vi "Page Log.vi"() -> ()   [LabVIEW 2018, in "Main.lvlib"]
uses:
  Main.lvlib
panel:
  out "current time":timestamp
  in  "Listbox":i32(listbox)=-1
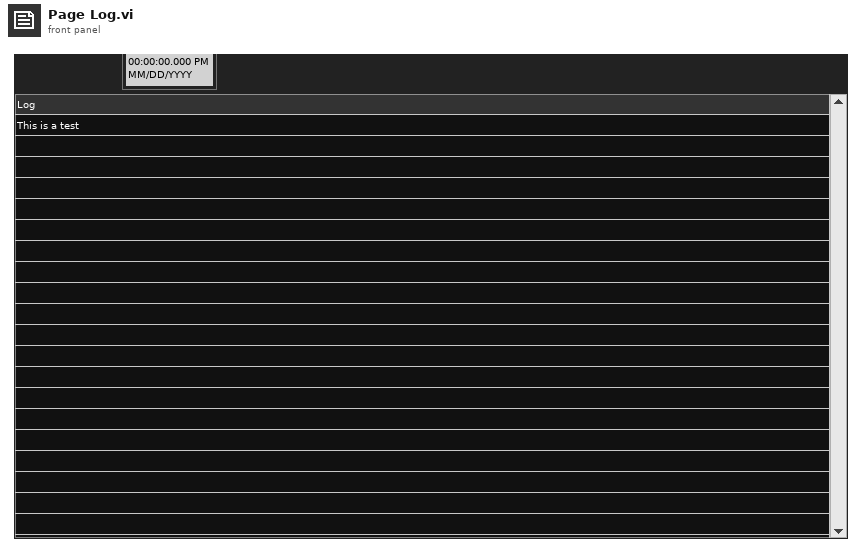
[diagram p1: front panel]
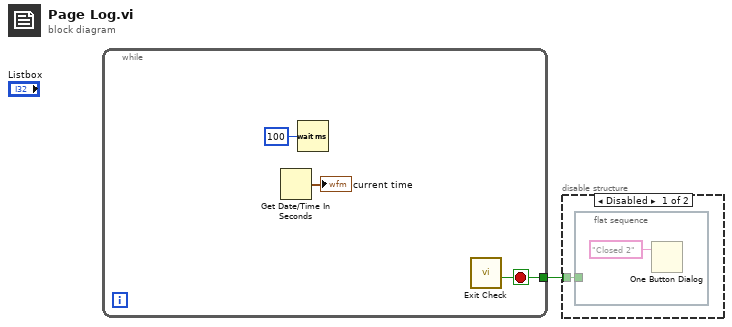
[diagram p0: block diagram]
diagram:
  n1 = while {
    tunnel: [w2] -> w1
    stop <- w2 stop-if-true
    n2 = Get Date/Time In Seconds() -> (seconds since 1Jan1904=→"current time":timestamp)
    n3 = Wait (ms)(milliseconds to wait=u32 100) -> ()  [unwired: 1 out]
    n4 = call "Exit Check.vi"() -> ("Exit?"=w2:bool)  [unwired: 10 in, 1 out]
  }
  n5 = disable-structure shown="Disabled" {
    disable-tunnel: w1 -> [w5 _]
    frame Disabled {
      n6 = flat-sequence {
        tunnel: w5 -> [_]
        frame #0 {
          n7 = One Button Dialog(message="Closed 2") -> ()  [unwired: 1 in, 1 out]
        }
      }
    }
    frame Enabled {
    }
  }
